vi "Envelope Data.vi"() -> ()   [LabVIEW 8.6]
uses:
  <vilib>/Analysis/NI_AALPro.lvlib
panel:
  in  "stop":bool
  out "appended array":waveform(dbl)[](graph)
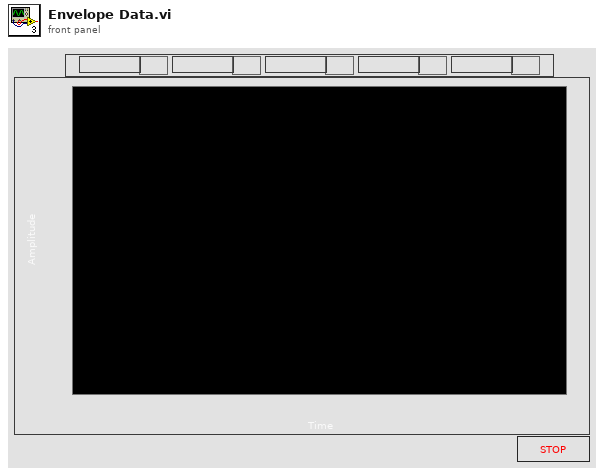
[diagram p1: front panel]
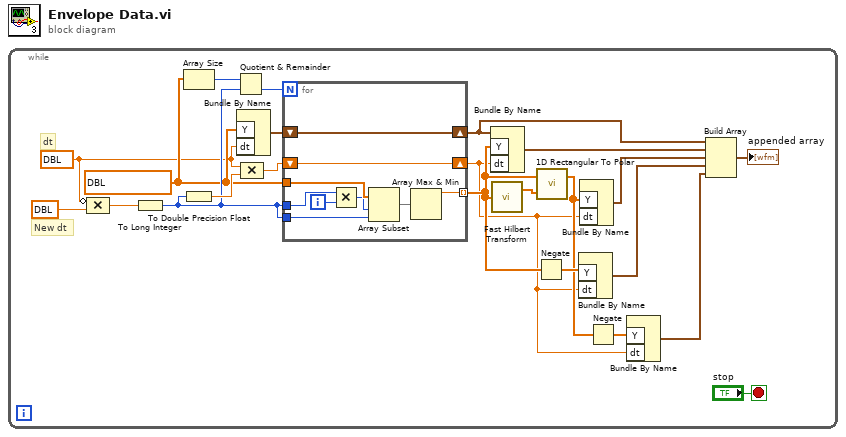
[diagram p0: block diagram]
diagram:
  n1 = while {
    stop <- "stop" stop-if-true
    w9 = dbl ? ("dt")
    w10 = dbl[] ? ("Y")
    # "New dt"
    # "dt"
    n2 = Compound Arithmetic op=MULTIPLY(invert w9, dbl ? ("New Value for dt")) -> (w19:dbl)
    n3 = To Long Integer(number=w19) -> (32bit integer=w15:i32)
    n4 = Array Size(array=w10) -> (size(s)=w21:i32)
    n5 = To Double Precision Float(number=w15) -> (double precision float=w16:dbl)
    n6 = Quotient & Remainder(x=w21, y=w15) -> (floor(x/y)=w18:i32)  [unwired: 1 out]
    n7 = Bundle By Name("Y"=w10, "dt"=w9) -> (w11:waveform(dbl))  [unwired: 1 in]
    n8 = Compound Arithmetic op=MULTIPLY(w9, w16) -> (w17:dbl)
    n9 = for {
      N: w18 -> [_]
      tunnel: w10 -> [w32]
      tunnel: w15 -> [w30]
      tunnel: w15 -> [w28]
      tunnel: [w26] -> w7 mode=indexing
      shift-right: [w25] -> w14
      shift-left: w11 -> [w25]
      shift-right: [w24] -> w3
      shift-left: w17 -> [w24]
      i -> [w31]
      n10 = Multiply(x=w30, y=w31) -> (x*y=w29:i32)
      n11 = Array Subset(array=w32, index=w29, length=w28) -> (w27:dbl[])
      n12 = Array Max & Min(array=w27) -> (max value=w26:dbl)  [unwired: 3 out]
    }
    n13 = Bundle By Name(cluster=w14, "Y"=w7, "dt"=w3) -> (w13:waveform(dbl))
    n14 = call <vilib>:"Fast Hilbert Transform.vi"("X"=w7) -> ("Hilbert{X}"=w22:dbl[])  [unwired: 1 out]
    n15 = Negate(x=w7) -> (-x=w6:dbl[])
    n16 = call <vilib>:"1D Rectangular To Polar.vi"("X"=w7, "Y"=w22) -> ("Magnitude"=w4:dbl[])  [unwired: 2 out]
    n17 = Bundle By Name("Y"=w6, "dt"=w3) -> (w2:waveform(dbl))  [unwired: 1 in]
    n18 = Bundle By Name("Y"=w4, "dt"=w3) -> (w12:waveform(dbl))  [unwired: 1 in]
    n19 = Negate(x=w4) -> (-x=w5:dbl[])
    n20 = Bundle By Name("Y"=w5, "dt"=w3) -> (w1:waveform(dbl))  [unwired: 1 in]
    n21 = Build Array(w14, w13, w12, w2, w1) -> (→"appended array":waveform(dbl)[])
  }
